vi "Config Folder Path-Switch.vi"(8 "error in (no error)":errorcluster) -> (0 "error out":errorcluster, 1 "file or folder exists?":bool, 2 "Development System":bool, 3 "dup path":path, 4 "Message string":string)   [LabVIEW 2017]
uses:
  <vilib>/Utility/config.llb/Read Key (Path).vi
  <vilib>/Utility/config.llb/Write Key (Path).vi
  <vilib>/Utility/config.llb/NI_LVConfig.lvlib
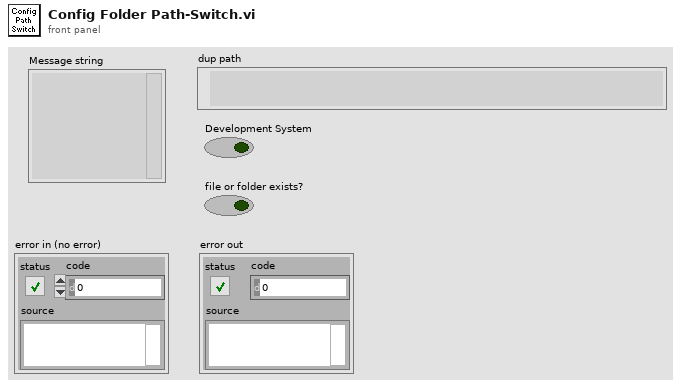
[diagram p1: front panel]
types:
  T1 = typedef "NI_LVConfig.lvlib/Config Data RefNum.ctl" = refnum<k1>
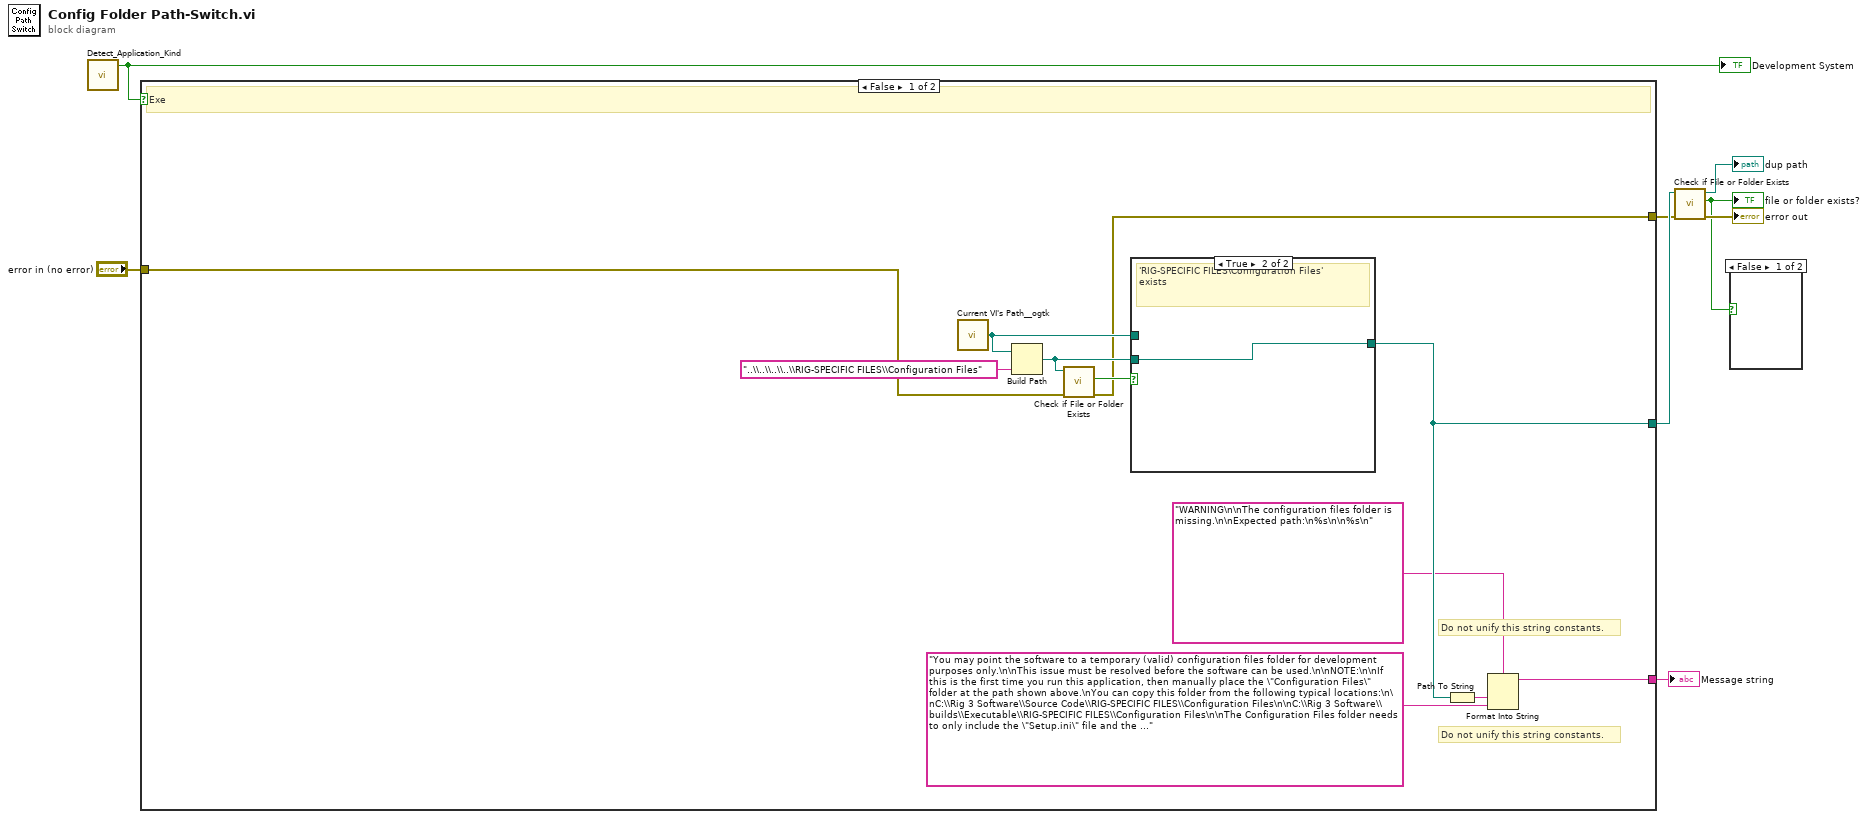
[diagram p0: block diagram]
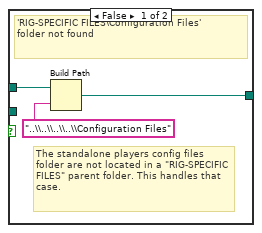
[diagram p3: hidden frame]
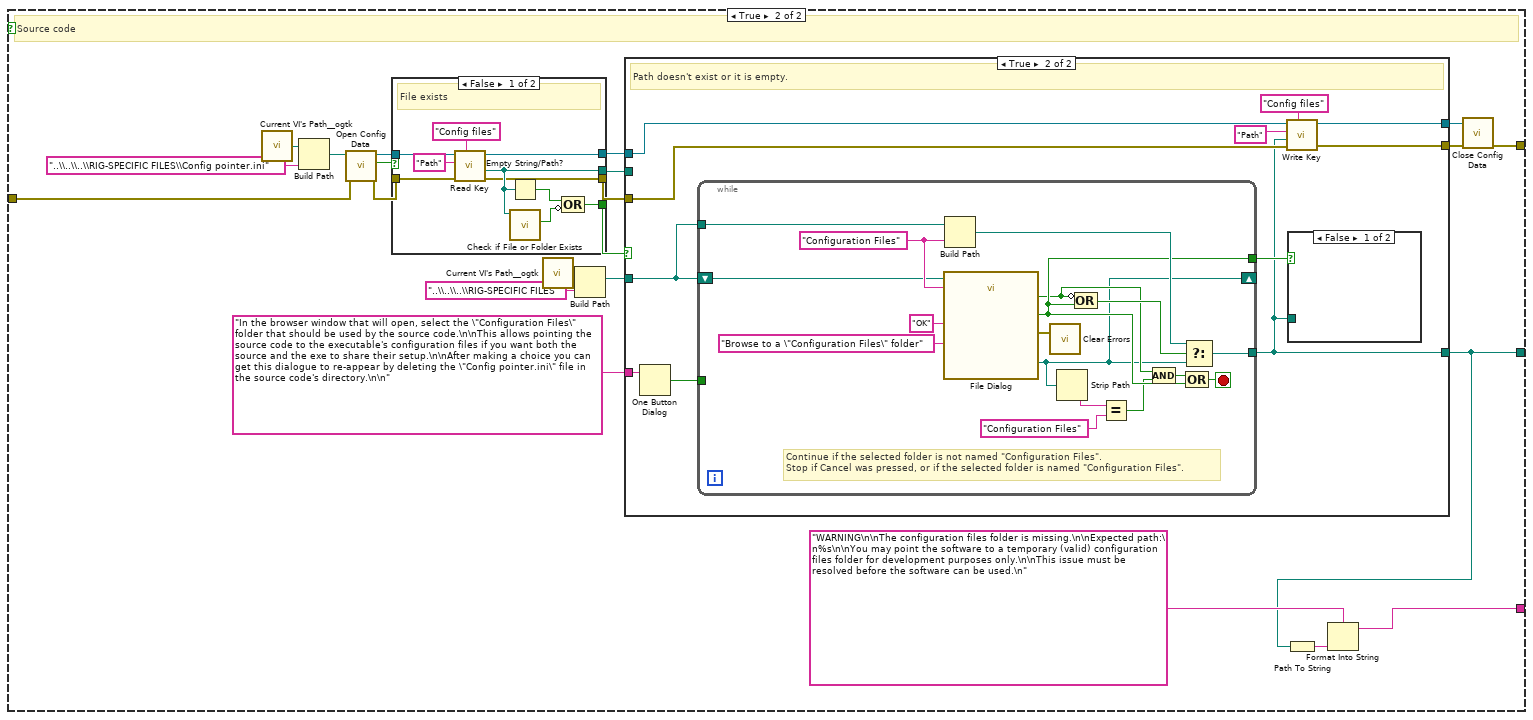
[diagram p4: hidden frame]
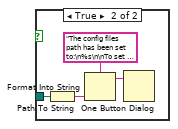
[diagram p6: hidden frame]
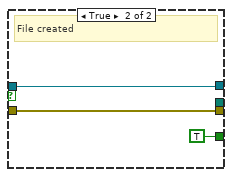
[diagram p7: hidden frame]
diagram:
  n1 = call <userlib>:"Detect_Application_Kind.vi"() -> ("Development System"=w6:bool)  [unwired: 9 in, 2 out]
  "Development System" <- w6
  n2 = case shown="False" w6 {
    tunnel: [w14 w24] -> w5
    tunnel: [w11 w33] -> w4
    tunnel: "error in (no error)" -> [w12 w32]
    tunnel: [w17 w26] -> w2
    frame False {
      # "Do not unify this string constants."
      # "Do not unify this string constants."
      # "Exe"
      n3 = call <userlib>:"Current VI's Path__ogtk.vi"() -> ("Current VI's Path (+ Relative)"=w13:path)  [unwired: 1 in]
      n4 = Build Path(base path=w13, name or relative path="..\\..\\..\\..\\RIG-SPECIFIC FILES\\Configuration Files") -> (appended path=w15:path)
      n5 = call <vilib>:"Check if File or Folder Exists.vi"("error in (no error)"=w12, "path"=w15) -> ("error out"=w11:errorcluster, "file or folder exists?"=w16:bool)  [unwired: 7 in, 1 out]
      n6 = case shown="True" w16 {
        tunnel: w15 -> [_ w23]
        tunnel: [w21 w23] -> w14
        tunnel: w13 -> [w22 _]
        frame False {
          # "The standalone players config files folder are not located in a \"RIG-SPECIFIC FILES\" parent folder. This handles that case."
          # "'RIG-SPECIFIC FILES\\Configuration Files' \nfolder not found"
          n7 = Build Path(base path=w22, name or relative path="..\\..\\..\\..\\Configuration Files") -> (appended path=w21:path)
        }
        frame True {
          # "'RIG-SPECIFIC FILES\\Configuration Files'\nexists"
        }
      }
      n8 = Path To String(path=w14) -> (string=w18:string)
      n9 = Format Into String(format string="WARNING\n\nThe configuration files folder is missing.\n\nExpected path:\n%s\n\n%s\n" ("Message string"), w18, "You may point the software to a temporary (valid) configuration files folder for development purposes only.\n\nThis issue must be resolved before the software can be used.\n\nNOTE:\n\nIf this is the first time you run this application, then manually place the \"Configuration Files\" folder at the path shown above.\nYou can copy this folder from the following typical locations:\n\nC:\\Rig 3 Software\\Source Code\\RIG-SPECIFIC FILES\\Configuration Files\n\nC:\\Rig 3 Software\\builds\\Executable\\RIG-SPECIFIC FILES\\Configuration Files\n\nThe Configuration Files folder needs to only include the \"Setup.ini\" file and the \"Default profile.ini\" inside its sub-folder. The rest of the files can be deleted.\n\nThe reason these files are missing is that the executable build-spec and the executable installer have been intentionally designed to NOT generate these configuration files, to avoid accidental overwrite of those files during software updates.\n" ("Message string")) -> (resulting string=w17:string)  [unwired: 2 in, 1 out]
    }
    frame True {
      # "Source code"
      n10 = call <userlib>:"Current VI's Path__ogtk.vi"() -> ("Current VI's Path (+ Relative)"=w45:path)  [unwired: 1 in]
      n11 = Build Path(base path=w45, name or relative path="..\\..\\..\\RIG-SPECIFIC FILES\\Config pointer.ini") -> (appended path=w43:path)
      n12 = call <vilib>:"Open Config Data.vi"("error in (no error)"=w32, "configuration file path"=w43) -> ("error out"=w41:errorcluster, "file created?"=w40:bool, "refnum"=w42:T1)  [unwired: 7 in]
      n13 = case shown="False" w40 {
        tunnel: w42 -> [w90 w93]
        tunnel: w41 -> [w89 w91]
        tunnel: [w86 _] -> w38
        tunnel: [w87 w93] -> w37
        tunnel: [w83 TRUE] -> w39
        tunnel: [w81 w91] -> w35
        frame False {
          # "File exists"
          n14 = call-poly <vilib>:"Read Key.vi"("section"="Config files", "error in (no error)"=w89, "key"="Path", "refnum"=w90) -> ("error out"=w81:errorcluster, "value"=w86:path, "refnum out"=w87:T1)  [unwired: 4 in, 1 out]
          n15 = Empty String/Path?(string/path=w86) -> (empty?=w84:bool)
          n16 = call <vilib>:"Check if File or Folder Exists.vi"("path"=w86) -> ("file or folder exists?"=w85:bool)  [unwired: 8 in, 2 out]
          n17 = Compound Arithmetic op=OR(w84, invert w85) -> (w83:bool)
        }
        frame True {
          # "File created"
        }
      }
      n18 = call <userlib>:"Current VI's Path__ogtk.vi"() -> ("Current VI's Path (+ Relative)"=w29:path)  [unwired: 1 in]
      n19 = Build Path(base path=w29, name or relative path="..\\..\\..\\RIG-SPECIFIC FILES") -> (appended path=w28:path)
      n20 = case shown="True" w39 {
        tunnel: w38 -> [w48 _]
        tunnel: [w48 w50] -> w24
        tunnel: w37 -> [w47 w58]
        tunnel: [w47 w57] -> w36
        tunnel: w35 -> [w46 w56]
        tunnel: [w46 w55] -> w34
        tunnel: "In the browser window that will open, select the \"Configuration Files\" folder that should be used by the source code.\n\nThis allows pointing the source code to the executable's configuration files if you want both the source and the exe to share their setup.\n\nAfter making a choice you can get this dialogue to re-appear by deleting the \"Config pointer.ini\" file in the source code's directory.\n\n" ("Message string") -> [_ w59]
        tunnel: w28 -> [_ w49]
        frame False {
          # "Path exists and it is valid"
        }
        frame True {
          # "Path doesn't exist or it is empty."
          n21 = One Button Dialog(message=w59) -> (true=w52:bool)  [unwired: 1 in]
          n22 = while {
            tunnel: w52 -> [_]
            tunnel: [w69] -> w51
            tunnel: [w76] -> w50
            shift-right: [w60] -> _
            shift-left: w49 -> [w62]
            tunnel: w49 -> [w61]
            stop <- w68 stop-if-true
            w73 = "Configuration Files" ("default name")
            # "Continue if the selected folder is not named \"Configuration Files\".\nStop if Cancel was pressed, or if the selected folder is named \"Configuration Files\"."
            n23 = call "File Dialog"("start path"=w62, "prompt"="Browse to a \"Configuration Files\" folder", "button label"="OK", "default name"=w73) -> ("selected path"=w60:path, "exists"=w67:bool, "cancelled"=w69:bool, "error out"=w74:errorcluster)  [unwired: 8 in]
            n24 = Build Path(base path=w61, name or relative path=w73) -> (appended path=w72:path)
            n25 = call <vilib>:"Clear Errors.vi"("error in (no error)"=w74) -> ()  [unwired: 5 in, 2 out]
            n26 = Strip Path(path=w60) -> (name=w65:string)  [unwired: 1 out]
            n27 = Compound Arithmetic op=OR(invert w67, w69) -> (w70:bool)
            n28 = Equal?(x=w65, y="Configuration Files" ("default name")) -> (x = y?=w63:bool)
            n29 = Compound Arithmetic op=AND(w67, w63) -> (w66:bool)
            n30 = Select(t=w72, s=w70, f=w60) -> (s? t:f=w76:path)
            n31 = Compound Arithmetic op=OR(w66, w69) -> (w68:bool)
          }
          n32 = call-poly <vilib>:"Write Key.vi"("section"="Config files", "error in (no error)"=w56, "value"=w50, "key"="Path", "refnum"=w58) -> ("error out"=w55:errorcluster, "refnum out"=w57:T1)  [unwired: 4 in, 1 out]
          n33 = case shown="False" w51 {
            tunnel: w50 -> [_ w78]
            frame False {
            }
            frame True {
              n34 = Path To String(path=w78) -> (string=w79:string)
              n35 = Format Into String(format string="The config files path has been set to:\n%s\n\nTo set a different path delete the \"Config pointer.ini\" file and restart the software." ("Message string"), w79) -> (resulting string=w80:string)  [unwired: 2 in, 1 out]
              n36 = One Button Dialog(message=w80) -> ()  [unwired: 1 in, 1 out]
            }
          }
        }
      }
      n37 = Path To String(path=w24) -> (string=w25:string)
      n38 = Format Into String(format string="WARNING\n\nThe configuration files folder is missing.\n\nExpected path:\n%s\n\nYou may point the software to a temporary (valid) configuration files folder for development purposes only.\n\nThis issue must be resolved before the software can be used.\n" ("Message string"), w25) -> (resulting string=w26:string)  [unwired: 2 in, 1 out]
      n39 = call <vilib>:"Close Config Data.vi"("error in (no error)"=w34, "refnum"=w36) -> ("error out"=w33:errorcluster)  [unwired: 8 in, 1 out]
    }
  }
  "Message string" <- w2
  n40 = call <vilib>:"Check if File or Folder Exists.vi"("error in (no error)"=w4, "path"=w5) -> ("error out"=→"error out":errorcluster, "file or folder exists?"=w1:bool, "dup path"=→"dup path":path)  [unwired: 7 in]
  "file or folder exists?" <- w1
  n41 = case shown="False" w1 {
    frame False {
    }
    frame True {
    }
  }
